vi "Is From Actor.vi"(11 "Sender in":refnum<class "Sender.lvclass">) -> (2 "Is From Actor":bool)   [LabVIEW 2020, in "jettl.lvlib" / "Sender.lvlib" / "Sender.lvclass"]
uses:
  Sender.lvclass
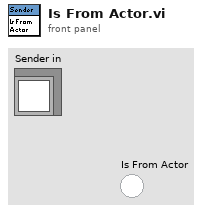
[diagram p1: front panel]
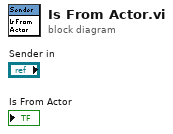
[diagram p0: block diagram]
diagram:
